vi "RTS Post Door Op Location.vi"(6 "System Number":T1="Select System", 8 "Error In":errorcluster, 9 "RTS Config Setup Input":T2, 11 "Search File Path Output":path) -> (0 "Error Out":errorcluster, 1 "RTS Config Setup Output":T2)   [LabVIEW 2020]
uses:
  Type Definitions/RTS Configuration Setup.ctl
  Type Definitions/RTS Wago Config.ctl
  Type Definitions/RTS APLUS Config.ctl
  Type Definitions/RTS Yokogawa MX Config.ctl
  Type Definitions/RTS Replay Server Control.ctl
  Type Definitions/RTS Server Configuration.ctl
  Type Definitions/RTS Station Settions TCP Comms.ctl
  Type Definitions/RTS Chamber Save Status.ctl
  Type Definitions/RTS Test Pattern.ctl
  Type Definitions/RTS Select System Number.ctl
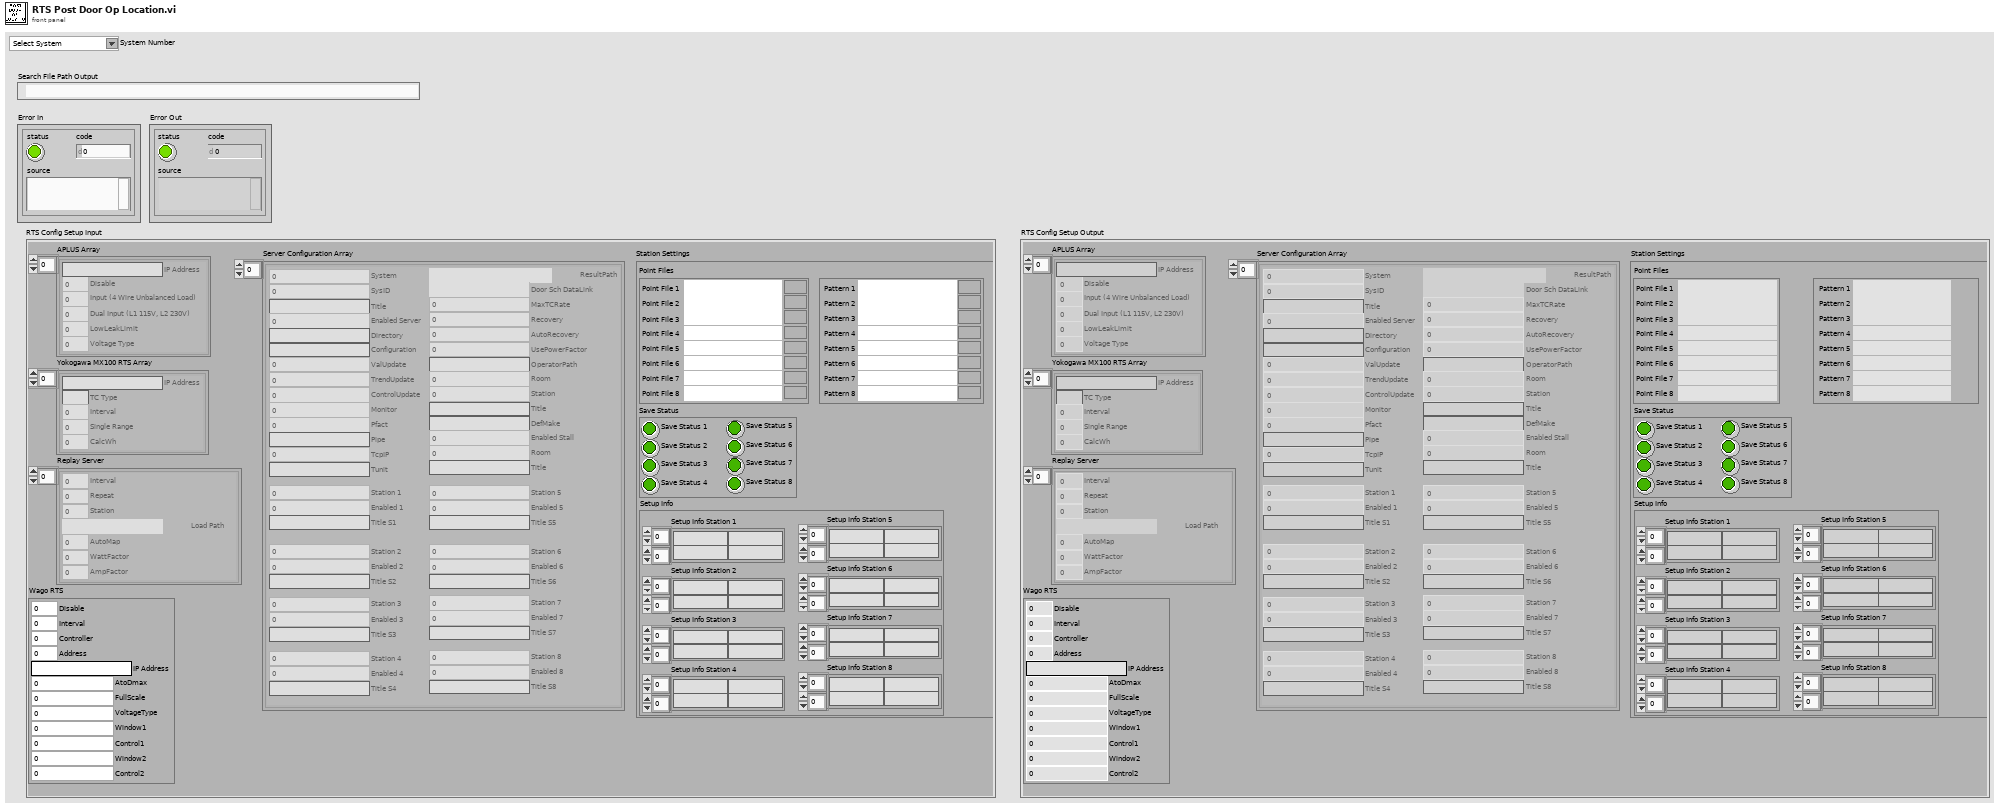
[diagram p1: front panel]
types:
  T1 = typedef "RTS Select System Number.ctl" = string
  T2 = typedef "RTS Configuration Setup.ctl" = cluster{"Wago RTS":T3, "APLUS Array":T4[], "Yokogawa MX100 RTS Array":T5[], "Replay Server":T6[], "Server Configuration Array":T7[], "Station Settings":T8}
  T3 = typedef "RTS Wago Config.ctl" = cluster{"Disable":u16, "Interval":u16, "Controller":u16, "Address":u16, "IP Address":string, "AtoDmax":u16, "FullScale":u16, "VoltageType":u16, "Window1":u16, "Control1":u16, "Window2":u16, "Control2":u16}
  T4 = typedef "RTS APLUS Config.ctl" = cluster{"Disable":u16, "IP Address":string, "Input (4 Wire Unbalanced Load)":u16, "Dual Input (L1 115V, L2 230V)":u16, "LowLeakLimit":dbl, "Voltage Type":u16}
  T5 = typedef "RTS Yokogawa MX Config.ctl" = cluster{"IP Address":string, "TC Type":string, "Interval":u16, "Single Range":u16, "CalcWh":u16}
  T6 = typedef "RTS Replay Server Control.ctl" = cluster{"Interval":i16, "Repeat":u16, "Station":u16, "Load Path":path, "AutoMap":u16, "WattFactor":dbl, "AmpFactor":dbl}
  T7 = typedef "RTS Server Configuration.ctl" = cluster{"System":u16, "SysID":u16, "Title":string, "Enabled Server":u16, "Directory":string, "Configuration":string, "ValUpdate":u16, "TrendUpdate":u16, "ControlUpdate":u16, "Monitor":u16, "Pfact":u16, "Pipe":string, "TcpIP":u16, "Tunit":string, "ResultPath":path, "Door Sch DataLink":path, "MaxTCRate":u16, "Recovery":u16, "AutoRecovery":u16, "UsePowerFactor":u16, "OperatorPath":string, "Room":u16, "Station":u16, "Title":string, "DefMake":string, "Enabled Stall":u16, "Room":u16, "Title":string, "Station 1":u16, "Enabled 1":u16, "Station 2":u16, "Enabled 2":u16, "Station 3":u16, "Enabled 3":u16, "Station 4":u16, "Enabled 4":u16, "Station 5":u16, "Enabled 5":u16, "Station 6":u16, "Enabled 6":u16, "Station 7":u16, "Enabled 7":u16, "Station 8":u16, "Enabled 8":u16, "Title S1":string, "Title S2":string, "Title S3":string, "Title S5":string, "Title S6":string, "Title S7":string, "Title S8":string, "Title S4":string}
  T8 = typedef "RTS Station Settions TCP Comms.ctl" = cluster{"Point Files":cluster{"Point File 1":path, "Point File 2":path, "Point File 3":path, "Point File 4":path, "Point File 5":path, "Point File 6":path, "Point File 7":path, "Point File 8":path}, "Save Status":T9, "Setup Info":cluster{"Setup Info Station 1":string[][], "Setup Info Station 2":string[][], "Setup Info Station 3":string[][], "Setup Info Station 4":string[][], "Setup Info Station 5":string[][], "Setup Info Station 6":string[][], "Setup Info Station 7":string[][], "Setup Info Station 8":string[][]}, "Chamber Test Pattern":T10}
  T9 = typedef "RTS Chamber Save Status.ctl" = cluster{"Save Status 1":bool, "Save Status 2":bool, "Save Status 3":bool, "Save Status 4":bool, "Save Status 5":bool, "Save Status 6":bool, "Save Status 7":bool, "Save Status 8":bool}
  T10 = typedef "RTS Test Pattern.ctl" = cluster{" Pattern 1":path, "Pattern 2":path, "Pattern 3":path, "Pattern 4":path, "Pattern 5":path, "Pattern 6":path, "Pattern 7":path, "Pattern 8":path}
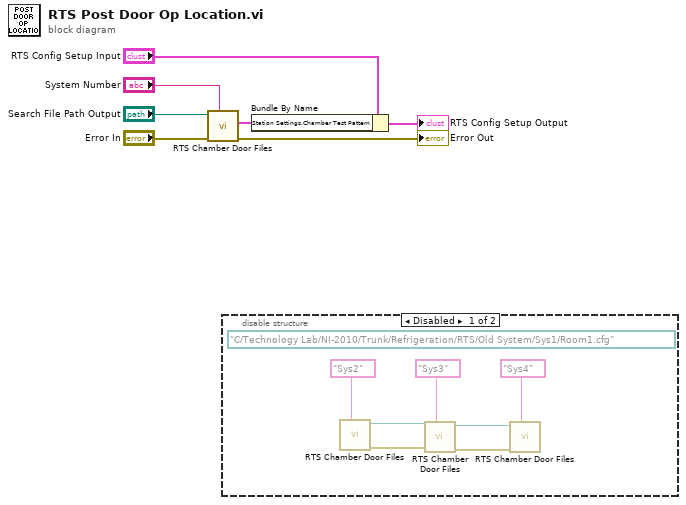
[diagram p0: block diagram]
diagram:
  n1 = call "RTS Chamber Door Files.vi"("System Number"="System Number", "error in (no error)"="Error In", "Search File Path Input"="Search File Path Output") -> ("error out"=→"Error Out":errorcluster, "Output"=w2:T10)  [unwired: 6 in, 1 out]
  n2 = disable-structure shown="Disabled" {
    frame Disabled {
      (unwired) path "C:/Technology Lab/NI-2010/Trunk/Refrigeration/RTS/Old System/Sys1/Room1.cfg" ("Search File Path Output")
      n3 = call "RTS Chamber Door Files.vi"("System Number"=T1 "Sys2") -> ("error out"=w14:errorcluster, "Search File Path Output"=w9:path)  [unwired: 8 in, 1 out]
      n4 = call "RTS Chamber Door Files.vi"("System Number"=T1 "Sys3", "error in (no error)"=w14, "Search File Path Input"=w9) -> ("error out"=w13:errorcluster, "Search File Path Output"=w8:path)  [unwired: 6 in, 1 out]
      n5 = call "RTS Chamber Door Files.vi"("System Number"=T1 "Sys4", "error in (no error)"=w13, "Search File Path Input"=w8) -> ()  [unwired: 6 in, 3 out]
    }
    frame Enabled {
    }
  }
  n6 = Bundle By Name(cluster="RTS Config Setup Input", "Station Settings.Chamber Test Pattern"=w2) -> (→"RTS Config Setup Output":T2)
